vi "Const_InitialChannels.vi"() -> (2 "appended array":string[][](array[string]))   [LabVIEW 2012]
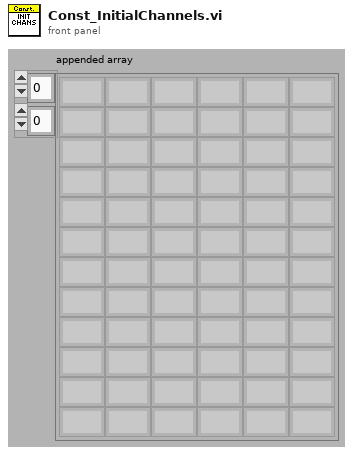
[diagram p1: front panel]
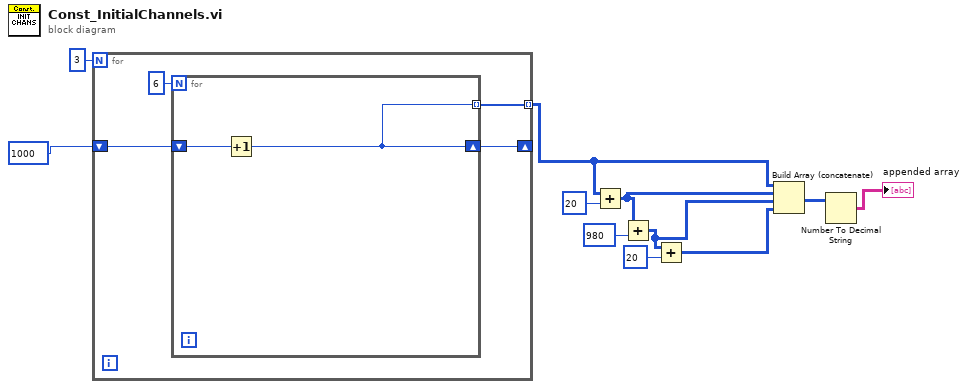
[diagram p0: block diagram]
diagram:
  n1 = for {
    N: 3 -> [_]
    shift-right: [w13] -> _
    shift-left: 1000 -> [w14]
    tunnel: [w12] -> w8 mode=indexing
    n2 = for {
      N: 6 -> [_]
      shift-right: [w16] -> w13
      shift-left: w14 -> [w17]
      tunnel: [w16] -> w12 mode=indexing
      n3 = Increment(x=w17) -> (x+1=w16:i32)
    }
  }
  n4 = Add(x=w8, y=20) -> (x+y=w6:i32[][])
  n5 = Add(x=w6, y=980) -> (x+y=w4:i32[][])
  n6 = Add(x=w4, y=20) -> (x+y=w3:i32[][])
  n7 = Build Array (concatenate)(w8, w6, w4, w3) -> (w2:i32[][])
  n8 = Number To Decimal String(number=w2) -> (decimal integer string=→"appended array":string[][])  [unwired: 1 in]
